vi "Actividad2.1.vi"() -> ()   [LabVIEW 2026]
panel:
  in  "stop":bool
  out "Tank 2":dbl(slide) scale=0.0..10.0
  out "Valvula Final":bool
  out "M":bool
  out "V1":bool
  in  "D_alto":bool
  in  "D_bajo":bool
  out "V2":bool
  in  "SP2":bool
  in  "SP1":bool
  out "VB":bool
  out "VA":bool
  out "Tank 1":dbl(slide) scale=0.0..10.0
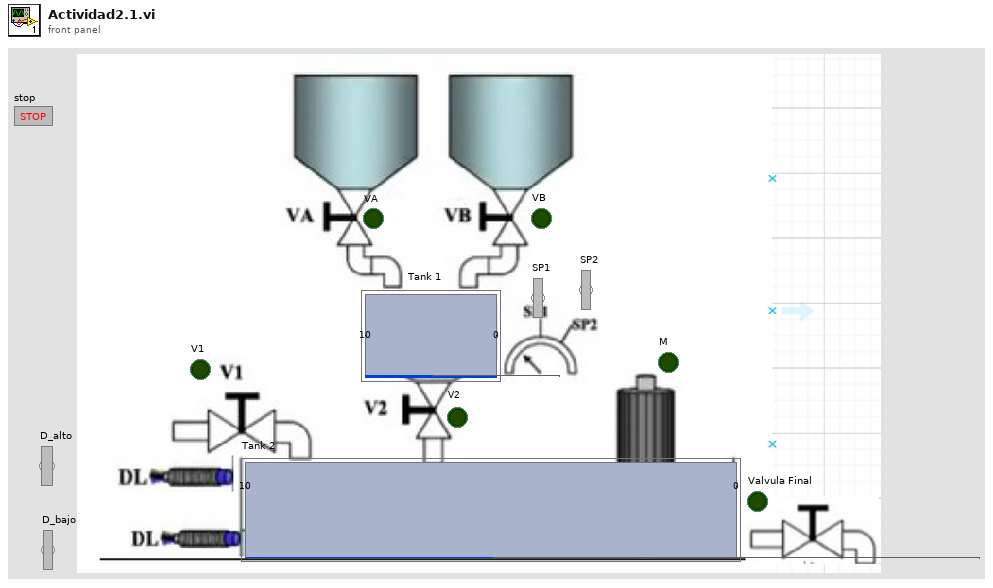
[diagram p1: front panel]
types:
  T1 = enum16{"Estado0", "Estado1", "Estado2", "Estado3", "Estado4", "Estado5", "Estado6", "Estado7", ""}
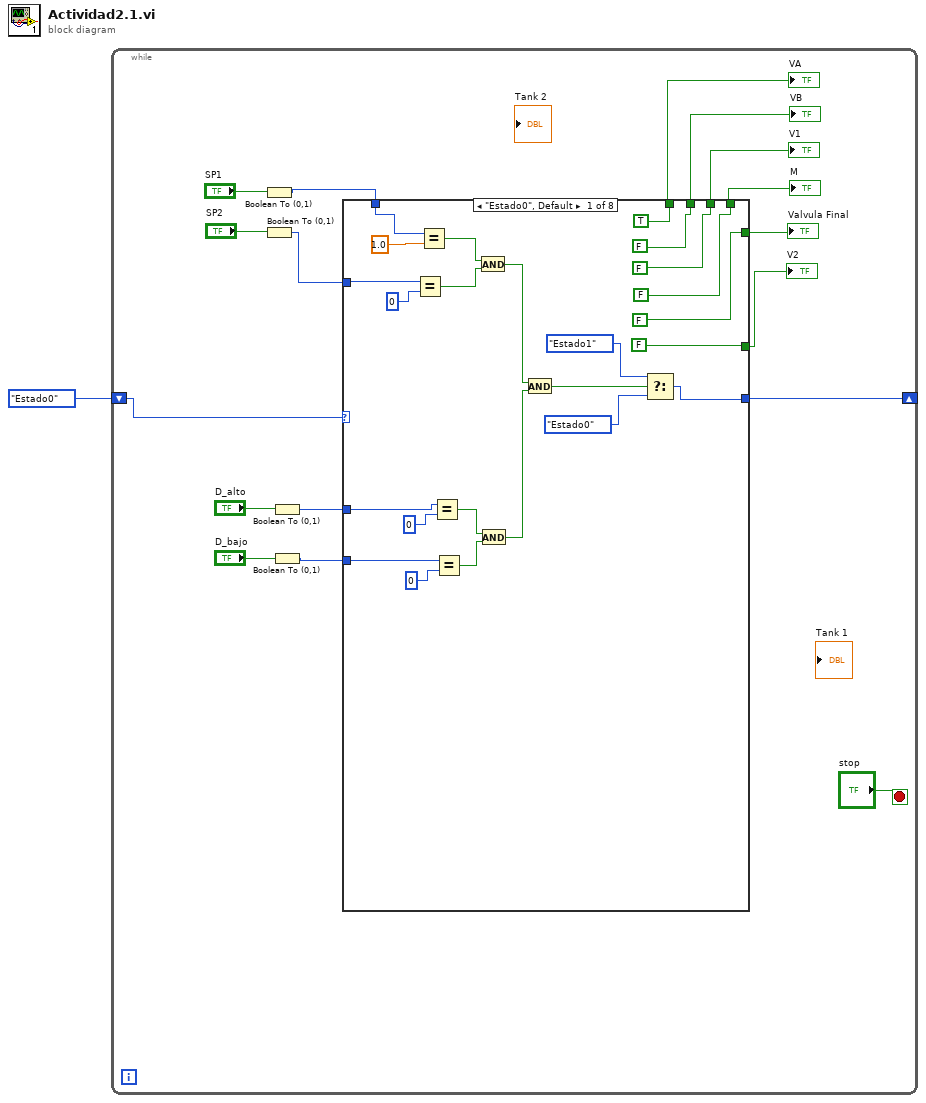
[diagram p0: block diagram]
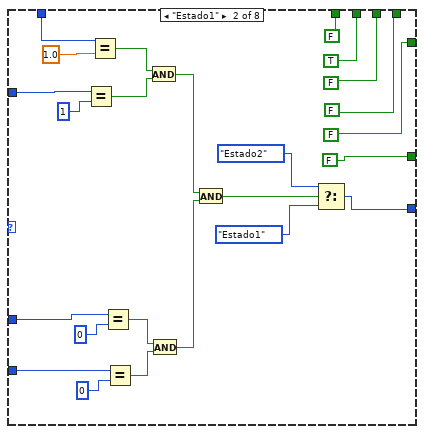
[diagram p2: hidden frame]
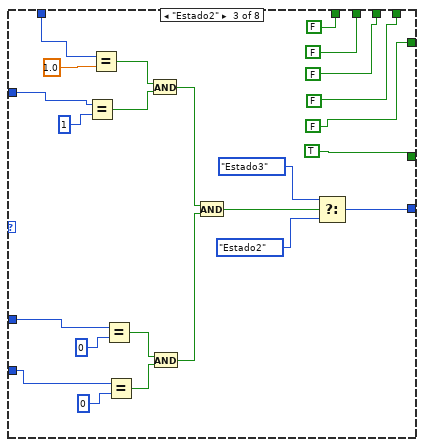
[diagram p3: hidden frame]
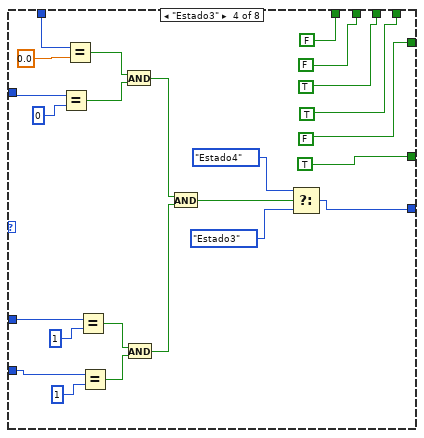
[diagram p4: hidden frame]
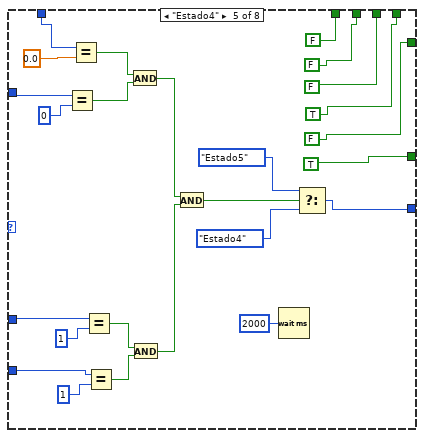
[diagram p5: hidden frame]
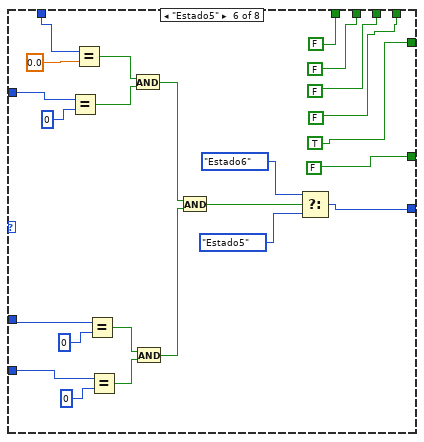
[diagram p6: hidden frame]
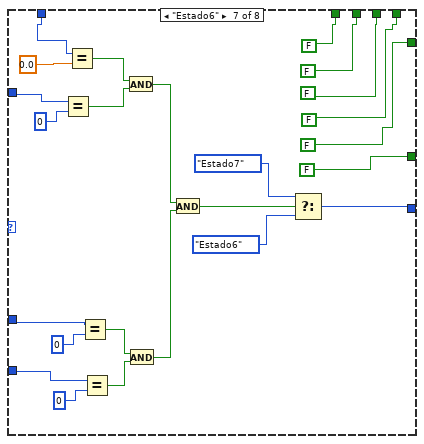
[diagram p7: hidden frame]
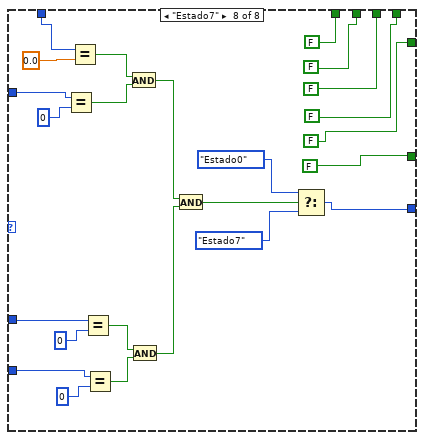
[diagram p8: hidden frame]
diagram:
  n1 = while {
    shift-right: [w2] -> _
    shift-left: T1."Estado0" -> [w17]
    stop <- "stop" stop-if-true
    n2 = Boolean To (0,1)(Boolean="SP1") -> (0, 1=w6:i16)
    n3 = Boolean To (0,1)(Boolean="SP2") -> (0, 1=w5:i16)
    n4 = Boolean To (0,1)(Boolean="D_alto") -> (0, 1=w4:i16)
    n5 = Boolean To (0,1)(Boolean="D_bajo") -> (0, 1=w3:i16)
    n6 = case shown="\"Estado0\", Default" w17 {
      tunnel: [TRUE FALSE FALSE FALSE FALSE FALSE FALSE FALSE] -> w16
      tunnel: [FALSE TRUE FALSE FALSE FALSE FALSE FALSE FALSE] -> w15
      tunnel: [FALSE FALSE FALSE TRUE FALSE FALSE FALSE FALSE] -> w14
      tunnel: [FALSE FALSE FALSE TRUE TRUE FALSE FALSE FALSE] -> w13
      tunnel: [FALSE FALSE FALSE FALSE FALSE TRUE FALSE FALSE] -> w12
      tunnel: [FALSE FALSE TRUE TRUE TRUE FALSE FALSE FALSE] -> w11
      tunnel: w6 -> [w29 w59 w76 w101 w126 w150 w174 w191]
      tunnel: w5 -> [w28 w58 w75 w100 w116 w149 w173 w190]
      tunnel: w4 -> [w27 w54 w74 w93 w125 w148 w172 w189]
      tunnel: w3 -> [w26 w53 w73 w92 w124 w147 w171 w188]
      tunnel: [w19 w43 w77 w91 w117 w140 w164 w192] -> w2
      frame "Estado0", Default {
        n7 = Equal?(x=w28, y=i16 0) -> (x = y?=w37:bool)
        n8 = Equal?(x=w29, y=1.0) -> (x = y?=w38:bool)
        n9 = Equal?(x=w27, y=i16 0) -> (x = y?=w36:bool)
        n10 = Equal?(x=w26, y=i16 0) -> (x = y?=w35:bool)
        n11 = And(x=w38, y=w37) -> (x .and. y?=w34:bool)
        n12 = And(x=w36, y=w35) -> (x .and. y?=w33:bool)
        n13 = And(x=w34, y=w33) -> (x .and. y?=w32:bool)
        n14 = Select(t=T1."Estado1", s=w32, f=T1."Estado0") -> (s? t:f=w19:T1)
      }
      frame "Estado1" {
        n15 = Equal?(x=w58, y=i16 1) -> (x = y?=w51:bool)
        n16 = Equal?(x=w59, y=1.0) -> (x = y?=w52:bool)
        n17 = Equal?(x=w54, y=i16 0) -> (x = y?=w50:bool)
        n18 = Equal?(x=w53, y=i16 0) -> (x = y?=w49:bool)
        n19 = And(x=w52, y=w51) -> (x .and. y?=w48:bool)
        n20 = And(x=w50, y=w49) -> (x .and. y?=w47:bool)
        n21 = And(x=w48, y=w47) -> (x .and. y?=w46:bool)
        n22 = Select(t=T1."Estado2", s=w46, f=T1."Estado1") -> (s? t:f=w43:T1)
      }
      frame "Estado2" {
        n23 = Equal?(x=w75, y=i16 1) -> (x = y?=w85:bool)
        n24 = Equal?(x=w76, y=1.0) -> (x = y?=w86:bool)
        n25 = Equal?(x=w74, y=i16 0) -> (x = y?=w84:bool)
        n26 = Equal?(x=w73, y=i16 0) -> (x = y?=w83:bool)
        n27 = And(x=w86, y=w85) -> (x .and. y?=w82:bool)
        n28 = And(x=w84, y=w83) -> (x .and. y?=w81:bool)
        n29 = And(x=w82, y=w81) -> (x .and. y?=w80:bool)
        n30 = Select(t=T1."Estado3", s=w80, f=T1."Estado2") -> (s? t:f=w77:T1)
      }
      frame "Estado3" {
        n31 = Equal?(x=w100, y=i16 0) -> (x = y?=w109:bool)
        n32 = Equal?(x=w101, y=0.0) -> (x = y?=w110:bool)
        n33 = Equal?(x=w93, y=i16 1) -> (x = y?=w108:bool)
        n34 = Equal?(x=w92, y=i16 1) -> (x = y?=w107:bool)
        n35 = And(x=w110, y=w109) -> (x .and. y?=w106:bool)
        n36 = And(x=w108, y=w107) -> (x .and. y?=w105:bool)
        n37 = And(x=w106, y=w105) -> (x .and. y?=w104:bool)
        n38 = Select(t=T1."Estado4", s=w104, f=T1."Estado3") -> (s? t:f=w91:T1)
      }
      frame "Estado4" {
        n39 = Equal?(x=w116, y=i16 0) -> (x = y?=w134:bool)
        n40 = Equal?(x=w126, y=0.0) -> (x = y?=w135:bool)
        n41 = Equal?(x=w125, y=i16 1) -> (x = y?=w133:bool)
        n42 = Equal?(x=w124, y=i16 1) -> (x = y?=w132:bool)
        n43 = And(x=w135, y=w134) -> (x .and. y?=w131:bool)
        n44 = And(x=w133, y=w132) -> (x .and. y?=w130:bool)
        n45 = And(x=w131, y=w130) -> (x .and. y?=w129:bool)
        n46 = Wait (ms)(milliseconds to wait=u32 2000) -> ()  [unwired: 1 out]
        n47 = Select(t=T1."Estado5", s=w129, f=T1."Estado4") -> (s? t:f=w117:T1)
      }
      frame "Estado5" {
        n48 = Equal?(x=w149, y=i16 0) -> (x = y?=w158:bool)
        n49 = Equal?(x=w150, y=0.0) -> (x = y?=w159:bool)
        n50 = Equal?(x=w148, y=i16 0) -> (x = y?=w157:bool)
        n51 = Equal?(x=w147, y=i16 0) -> (x = y?=w156:bool)
        n52 = And(x=w159, y=w158) -> (x .and. y?=w155:bool)
        n53 = And(x=w157, y=w156) -> (x .and. y?=w154:bool)
        n54 = And(x=w155, y=w154) -> (x .and. y?=w153:bool)
        n55 = Select(t=T1."Estado6", s=w153, f=T1."Estado5") -> (s? t:f=w140:T1)
      }
      frame "Estado6" {
        n56 = Equal?(x=w173, y=i16 0) -> (x = y?=w182:bool)
        n57 = Equal?(x=w174, y=0.0) -> (x = y?=w183:bool)
        n58 = Equal?(x=w172, y=i16 0) -> (x = y?=w181:bool)
        n59 = Equal?(x=w171, y=i16 0) -> (x = y?=w180:bool)
        n60 = And(x=w183, y=w182) -> (x .and. y?=w179:bool)
        n61 = And(x=w181, y=w180) -> (x .and. y?=w178:bool)
        n62 = And(x=w179, y=w178) -> (x .and. y?=w177:bool)
        n63 = Select(t=T1."Estado7", s=w177, f=T1."Estado6") -> (s? t:f=w164:T1)
      }
      frame "Estado7" {
        n64 = Equal?(x=w190, y=i16 0) -> (x = y?=w206:bool)
        n65 = Equal?(x=w191, y=0.0) -> (x = y?=w207:bool)
        n66 = Equal?(x=w189, y=i16 0) -> (x = y?=w205:bool)
        n67 = Equal?(x=w188, y=i16 0) -> (x = y?=w204:bool)
        n68 = And(x=w207, y=w206) -> (x .and. y?=w203:bool)
        n69 = And(x=w205, y=w204) -> (x .and. y?=w202:bool)
        n70 = And(x=w203, y=w202) -> (x .and. y?=w201:bool)
        n71 = Select(t=T1."Estado0", s=w201, f=T1."Estado7") -> (s? t:f=w192:T1)
      }
    }
    "VA" <- w16
    "VB" <- w15
    "V2" <- w11
    "V1" <- w14
    "M" <- w13
    "Valvula Final" <- w12
  }
